vi "Initialize.vi"(8 "error in (no error)":errorcluster, 9 "Reset (True)":bool, 10 "ID Query (True)":bool=TRUE, 11 "VISA resource name":refnum<visa-resource-name>) -> (0 "error out":errorcluster, 2 "ID":string, 3 "VISA resource name out":refnum<visa-resource-name>)   [LabVIEW 2020, in "QuPMXdriver.lvlib"]
doc: "Establishes communication with the instrument and optionally performs an instrument identification query and/or an instrument reset. It also places the instrument in a default state needed for other instrument driver operations. Therefore, call this VI before calling other instrument driver VIs for this instrument. Generally, you need to call the <b>Initialize</b> VI only once at the beginning of an application."
uses:
  QuPMXdriver.lvlib
panel:
  # "(c) 2021 Czech Metrology Institute.  ALL RIGHTS RESERVED."
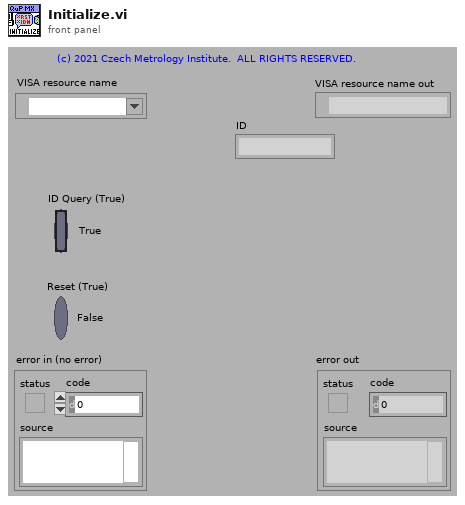
[diagram p1: front panel]
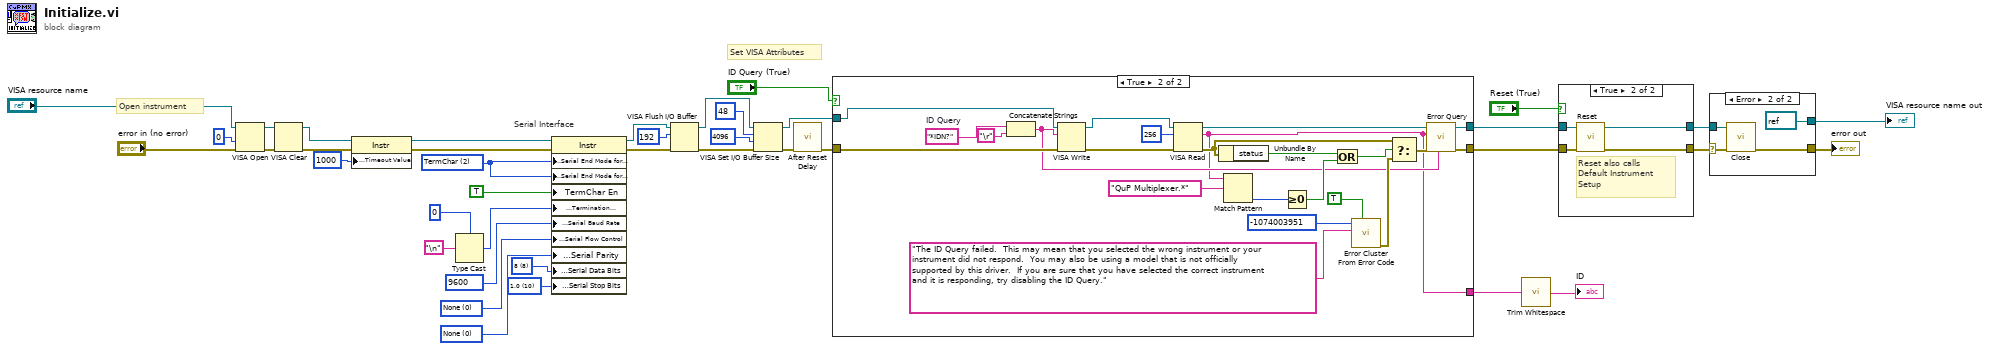
[diagram p0: block diagram]
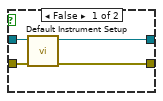
[diagram p3: hidden frame]
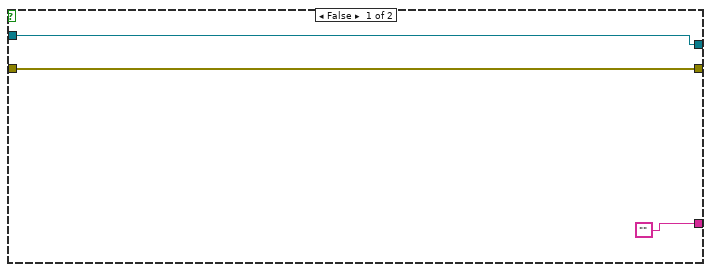
[diagram p4: hidden frame]
diagram:
  w10 = u32 9600 items=["300"=300, "600"=600, "1200"=1200, "2400"=2400, "4800"=4800, "9600"=9600, "19200"=19200] ("Baud Rate")
  w6 = u16 0 items=["None", "Odd", "Even", "Mark", "Space"] ("Parity")
  w9 = u16 8 items=["7"=7, "8"=8] ("Data Bits")
  w8 = u16 10 items=["1.0"=10, "1.5"=15, "2.0"=20] ("Stop Bits")
  w7 = u16 0 items=["None", "XON/XOFF", "RTS/CTS", "XON/XOFF & RTS/CTS", "DTR/DSR", "XON/XOFF & DTR/DSR"] ("Flow Control")
  w12 = u16 2 items=["None", "LastBit", "TermChar"] ("Serial Settings:Serial End Mode for Reads")
  # "Serial Interface"
  # "Set VISA Attributes"
  # "Open instrument"
  n1 = VISA Open(access mode=u32 0, error in (no error)="error in (no error)", VISA resource name="VISA resource name") -> (VISA resource name=w29:refnum<visa-resource-name>, error out=w28:errorcluster)  [unwired: 2 in]
  n2 = VISA Clear(VISA resource name=w29, error in (no error)=w28) -> (VISA resource name out=w27:refnum<visa-resource-name>, error out=w26:errorcluster)
  n3 = property class="Instr"(reference=w27, error in=w26, "General Settings:Timeout Value"=u32 1000) -> (reference out=w32:refnum<visa-resource-name>, error out=w31:errorcluster)
  n4 = Type Cast(type=u8 0, x="\n" ("Line Feed Constant")) -> (*(type *) &x=w11:u8)
  n5 = property class="Instr"(reference=w32, error in=w31, "Serial Settings:Serial End Mode for Reads"=w12, "Serial Settings:Serial End Mode for Writes"=w12, "TermChar En"=TRUE ("Message Based Settings:Termination Character Enable"), "Message Based Settings:Termination Character"=w11, "Serial Settings:Serial Baud Rate"=w10, "Serial Settings:Serial Flow Control"=w7, "Serial Settings:Serial Parity"=w6, "Serial Settings:Serial Data Bits"=w9, "Serial Settings:Serial Stop Bits"=w8) -> (reference out=w18:refnum<visa-resource-name>, error out=w20:errorcluster)
  n6 = VISA Flush I/O Buffer(VISA resource name=w18, mask (16)=u16 192, error in (no error)=w20) -> (VISA resource name out=w21:refnum<visa-resource-name>, error out=w19:errorcluster)
  n7 = VISA Set I/O Buffer Size(VISA resource name=w21, mask (16)=u16 48, size (4096)=u32 4096 ("size (0)"), error in (no error)=w19) -> (VISA resource name out=w33:refnum<visa-resource-name>, error out=w4:errorcluster)
  n8 = call "After Reset Delay.vi"("error in"=w4) -> ("error out"=w3:errorcluster)  [unwired: 10 in]
  n9 = case shown="True" "ID Query (True)" {
    tunnel: [w42 w49] -> w39
    tunnel: [w43 w48] -> w40
    tunnel: w33 -> [w43 w65]
    tunnel: w3 -> [w42 w66]
    tunnel: ["" w45] -> w2
    frame False {
    }
    frame True {
      w51 = "*IDN?"  # ID Query
      n10 = Concatenate Strings(w51, "\r") -> (w46:string)
      n11 = VISA Write(VISA resource name=w65, write buffer=w46, error in (no error)=w66) -> (VISA resource name out=w64:refnum<visa-resource-name>, error out=w44:errorcluster)  [unwired: 1 out]
      n12 = VISA Read(VISA resource name=w64, byte count=u32 256, error in (no error)=w44) -> (VISA resource name out=w47:refnum<visa-resource-name>, read buffer=w45:string, error out=w56:errorcluster)  [unwired: 1 out]
      n13 = Unbundle By Name(w56) -> ("status"=w55:bool)
      n14 = Match Pattern(string=w45, regular expression="QuP Multiplexer.*") -> (offset past match=w57:i32)  [unwired: 1 in, 3 out]
      n15 = Greater Or Equal To 0?(x=w57) -> (x >= 0?=w54:bool)
      n16 = Or(x=w55, y=w54) -> (x .or. y?=w53:bool)
      n17 = call <vilib>:"Error Cluster From Error Code.vi"("show call chain? (False)"=TRUE, "error message (\"\")"="The ID Query failed.  This may mean that you selected the wrong instrument or your instrument did not respond.  You may also be using a model that is not officially supported by this driver.  If you are sure that you have selected the correct instrument and it is responding, try disabling the ID Query." ("Source (VI Name)"), "error code (0)"=-1074003951 ("Code")) -> ("error out"=w61:errorcluster)  [unwired: 6 in]
      n18 = Select(t=w56, s=w53, f=w61) -> (s? t:f=w50:errorcluster)
      n19 = call "Error Query.vi"("Last command"=w46, "error in (no error)"=w50, "Read buffer"=w45, "VISA resource name"=w47) -> ("error out"=w49:errorcluster, "VISA resource name out"=w48:refnum<visa-resource-name>)  [unwired: 6 in]
    }
  }
  n20 = call <vilib>:"Trim Whitespace.vi"("string"=w2) -> ("trimmed string"=→"ID":string)  [unwired: 1 in]
  n21 = case shown="True" "Reset (True)" {
    tunnel: w39 -> [w69 w71]
    tunnel: [w67 w74] -> w22
    tunnel: w40 -> [w70 w72]
    tunnel: [w68 w73] -> w23
    frame False {
      n22 = call "Default Instrument Setup.vi"("error in (no error)"=w69, "VISA resource name"=w70) -> ("error out"=w67:errorcluster, "VISA resource name out"=w68:refnum<visa-resource-name>)  [unwired: 8 in]
    }
    frame True {
      # "Reset also calls Default Instrument Setup"
      n23 = call "Reset.vi"("error in (no error)"=w71, "VISA resource name"=w72) -> ("error out"=w74:errorcluster, "VISA resource name out"=w73:refnum<visa-resource-name>)  [unwired: 8 in]
    }
  }
  n24 = case shown="Error" w22 {
    selector: w22 -> [w75 w78]
    tunnel: w23 -> [w76 w79]
    tunnel: [w76 refnum<visa-resource-name> refnum ("VISA resource name out")] -> w25
    tunnel: [w75 w80] -> w24
    frame No Error {
    }
    frame Error {
      n25 = call "Close.vi"("error in (no error)"=w78, "VISA resource name"=w79) -> ("error out"=w80:errorcluster)  [unwired: 9 in]
    }
  }
  "VISA resource name out" <- w25
  "error out" <- w24
